vi "Write FPGA Channel Setting.vi"(8 "error in (no error)":errorcluster, 10 "FPGA Channel Setting":T1={"Numeric"=0.5, "Combo"="", "String"="", "Boolean"=FALSE} {"Numeric" format="%#_f"}, 11 "Channel configuration in":refnum<class "FPGA Channel configuration.lvclass">) -> (0 "error out":errorcluster, 3 "Channel configuration out":refnum<class "FPGA Channel configuration.lvclass">)   [LabVIEW 2025, in "FPGA.lvlib" / "FPGA Channel configuration.lvclass"]
uses:
  FPGA Channel configuration.lvclass
  FPGA Channel Setting.ctl
  FPGA Channel configuration.lvclass/FPGA Channel configuration.ctl
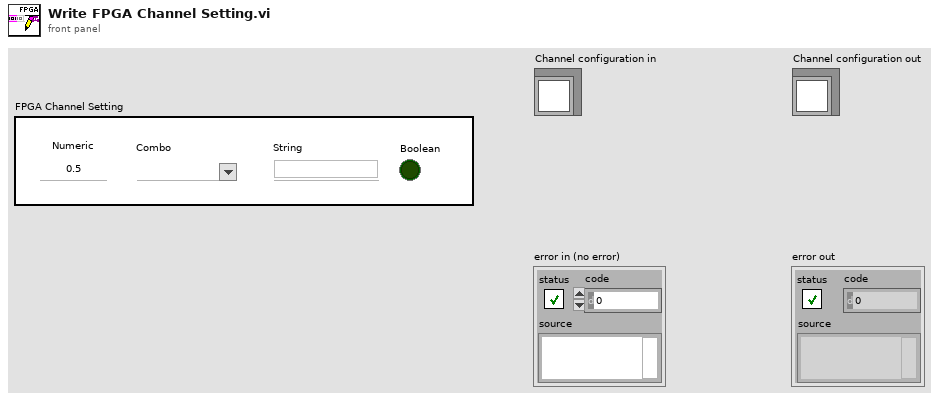
[diagram p1: front panel]
types:
  T1 = typedef "FPGA.lvlib/FPGA Channel configuration.lvclass/FPGA Channel Setting.ctl" = cluster{"Numeric":dbl, "Combo":string, "String":string, "Boolean":bool}
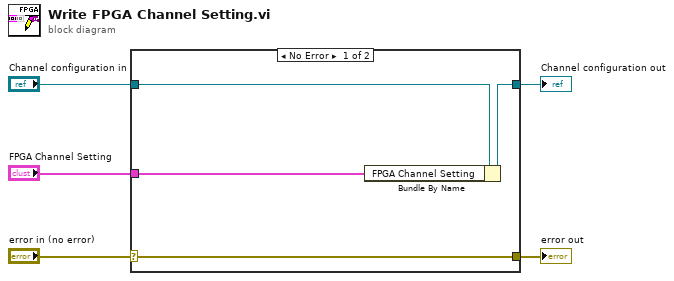
[diagram p0: block diagram]
diagram:
  n1 = case shown="No Error" "error in (no error)" {
    selector: "error in (no error)" -> [w9 w10]
    tunnel: [w9 w10] -> w4
    tunnel: [w7 w11] -> w2
    tunnel: "Channel configuration in" -> [w8 w11]
    tunnel: "FPGA Channel Setting" -> [w6 _]
    frame No Error {
      n2 = Bundle By Name(cluster=w8, "FPGA Channel Setting"=w6) -> (w7:refnum<class "FPGA Channel configuration.lvclass">)
    }
    frame Error {
    }
  }
  "error out" <- w4
  "Channel configuration out" <- w2
